vi "Load.vi"(8 "error in (no error)":errorcluster, 10 "File":path, 11 "SPXMusicLibrary in":refnum<class "SPXMusicLibrary.lvclass">) -> (0 "error out":errorcluster, 3 "SPXMusicLibrary out":refnum<class "SPXMusicLibrary.lvclass">)   [LabVIEW 2015, in "SPXMusicLibrary.lvclass"]
uses:
  SPXMusicLibrary.lvclass
  src/file/MusicElement/MusicElementLibrary/MusicLibrary/MusicLibrary.lvclass
  src/file/MusicElement/Song/Song.lvclass
  src/file/MusicElement/MusicFile/MusicFile.lvclass/MusicFile.ctl
  <vilib>/Utility/file.llb/Read Delimited Spreadsheet (string).vi
  src/file/MusicElement/Album/Album.lvclass
  src/file/MusicElement/MusicElementLibrary/MusicElementLibrary.lvclass
  src/file/MusicElement/MusicFile/MusicFile.lvclass
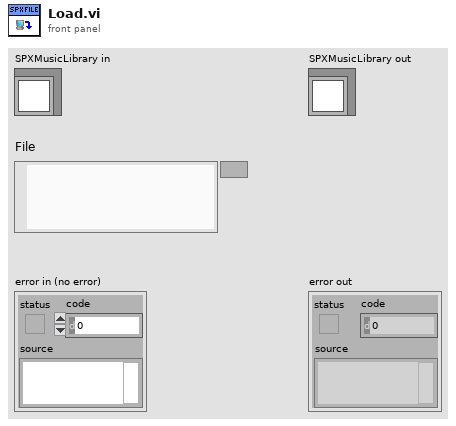
[diagram p1: front panel]
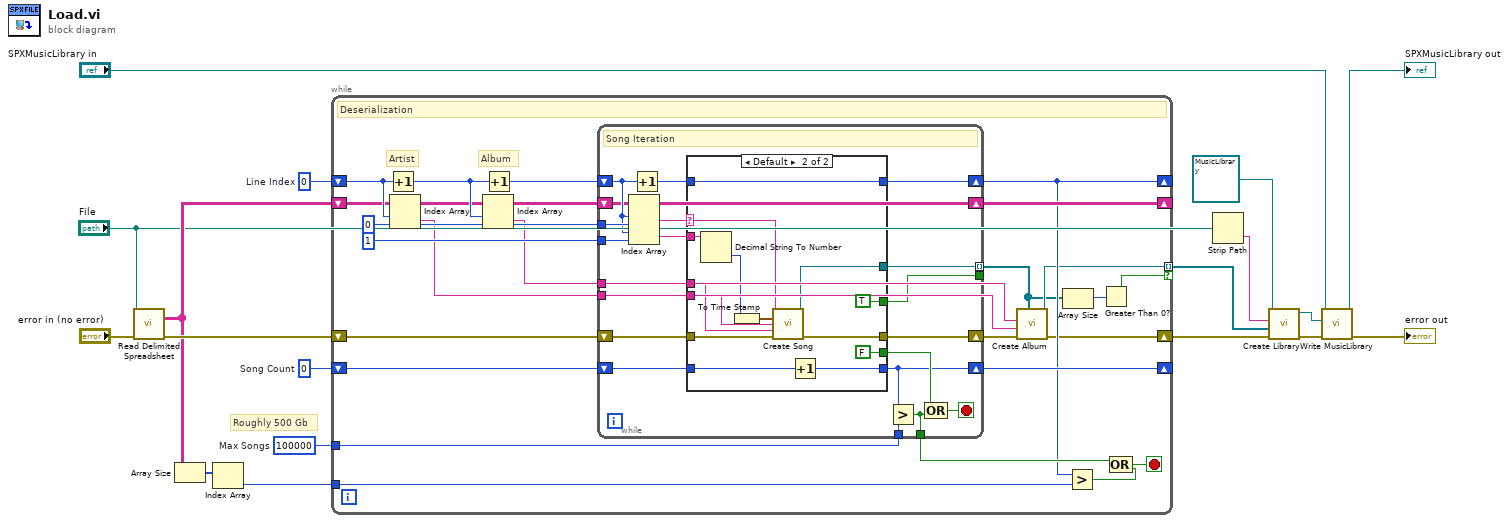
[diagram p0: block diagram]
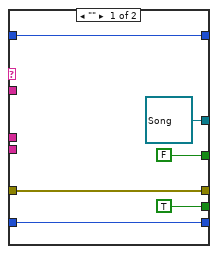
[diagram p2: hidden frame]
diagram:
  w15 = 0  # Song Count
  w14 = 100000  # Max Songs
  w16 = 0  # Line Index
  # "Roughly 500 Gb"
  n1 = call-poly <vilib>:"Read Delimited Spreadsheet.vi"("file path (dialog if empty)"="File", "error in (no error)"="error in (no error)") -> ("all rows"=w13:string[][], "error out"=w17:errorcluster)  [unwired: 8 in, 4 out]
  n2 = Array Size(array=w13) -> (size(s)=w12:i32[])
  n3 = Index Array(array=w12) -> (element=w11:i32)  [unwired: 1 in]
  n4 = while {
    shift-right: [w19] -> w6
    shift-left: w17 -> [w27]
    shift-right: [w34] -> _
    shift-left: w13 -> [w38]
    shift-right: [w30] -> _
    shift-left: w16 -> [w42]
    tunnel: w14 -> [w36]
    shift-right: [w35] -> _
    shift-left: w15 -> [w41]
    tunnel: w11 -> [w29]
    tunnel: [w23] -> w5 mode=indexing if=w20
    stop <- w32 stop-if-true
    w33 = 0 ("disabled index (col)")
    # "Album"
    # "Artist"
    # "Deserialization"
    n5 = Increment(x=w42) -> (x+1=w40:i32)
    n6 = Index Array(array=w38, index (row)=w42, index (col)=w33) -> (element=w24:string)
    n7 = Index Array(array=w38, index (row)=w40, index (col)=w33) -> (element=w25:string)
    n8 = Increment(x=w40) -> (x+1=w39:i32)
    n9 = while {
      shift-right: [w54] -> w30
      shift-left: w39 -> [w57]
      shift-right: [w45] -> w26
      shift-left: w27 -> [w62]
      shift-right: [w49] -> w34
      shift-left: w38 -> [w49]
      tunnel: w33 -> [w60]
      tunnel: 1 ("disabled index (col)") -> [w59]
      tunnel: w36 -> [w53]
      tunnel: [w52] -> w31
      shift-right: [w48] -> w35
      shift-left: w41 -> [w61]
      tunnel: w25 -> [w46]
      tunnel: w24 -> [w47]
      tunnel: [w44] -> w22 mode=indexing if=w43
      tunnel: [w43] -> _
      stop <- w50 stop-if-true
      # "Song Iteration"
      n10 = Index Array(array=w49, index (row) #1=w57, index (col) #1=w60, index (row) #2=w57, index (col) #2=w59) -> (element #1=w58:string, element #2=w56:string)
      n11 = Increment(x=w57) -> (x+1=w55:i32)
      n12 = case shown="Default" w58 {
        selector: w58 -> [_ w79]
        tunnel: [w68 w73] -> w45
        tunnel: [refnum<class "Song.lvclass"> refnum ("Song out") w70] -> w44
        tunnel: w62 -> [w68 w82]
        tunnel: w61 -> [w65 w81]
        tunnel: w56 -> [_ w80]
        tunnel: w55 -> [w67 w78]
        tunnel: [w67 w78] -> w54
        tunnel: [w65 w77] -> w48
        tunnel: [TRUE ("value") FALSE ("value")] -> w51
        tunnel: w47 -> [_ w72]
        tunnel: w46 -> [_ w71]
        tunnel: [FALSE ("value") TRUE ("value")] -> w43
        frame "" {
        }
        frame Default {
          n13 = Decimal String To Number(string=w80) -> (number=w75:i32)  [unwired: 2 in, 1 out]
          n14 = To Time Stamp(1:w75) -> (0:w74:timestamp)
          n15 = call "Create Song.vi"("Name"=w79, "Duration (s)"=w74, "Artist"=w72, "Album"=w71, "error in (no error)"=w82) -> ("Song out"=w70:refnum<class "Song.lvclass">, "error out"=w73:errorcluster)  [unwired: 9 in]
          n16 = Increment(x=w81) -> (x+1=w77:i32)
        }
      }
      n17 = Greater?(x=w48, y=w53) -> (0:w52:bool)
      n18 = Compound Arithmetic op=OR(w51, w52) -> (w50:bool)
    }
    n19 = call "Create Album.vi"("Songs"=w22, "error in (no error)"=w26, "Artist Name"=w24, "Album Name"=w25) -> ("error out"=w19:errorcluster, "Album out"=w23:refnum<class "Album.lvclass">)  [unwired: 6 in]
    n20 = Array Size(array=w22) -> (size(s)=w21:i32)
    n21 = Greater?(x=w30, y=w29) -> (0:w28:bool)
    n22 = Greater Than 0?(x=w21) -> (x > 0?=w20:bool)
    n23 = Compound Arithmetic op=OR(w31, w28) -> (w32:bool)
  }
  n24 = Strip Path(path="File") -> (name=w9:string)  [unwired: 1 out]
  n25 = call "Create Library.vi"("error in (no error)"=w6, "Music Element Library"=w5, "Name"=w9, "MusicElementLibrary in"=refnum<class "MusicLibrary.lvclass"> refnum ("MusicLibrary.lvclass")) -> ("error out"=w7:errorcluster, "MusicElementLibrary out"=w3:refnum<class "MusicLibrary.lvclass">)  [unwired: 6 in]
  n26 = call "Write MusicLibrary.vi"("error in (no error)"=w7, "MusicLibrary.lvclass"=w3, "MusicFile in"="SPXMusicLibrary in") -> ("error out"=→"error out":errorcluster, "MusicFile out"=→"SPXMusicLibrary out":refnum<class "SPXMusicLibrary.lvclass">)  [unwired: 7 in]
